vi "PID_2021.vi"(4 "Reset":bool, 5 "Lower limit":dbl, 6 "dt (s)":dbl, 7 "Upper limit":dbl, 8 "Setpoint":dbl, 9 "Process Variable":dbl, 10 "PID gains":cluster{"Kp":dbl, "Ki":dbl, "Kd":dbl}) -> (2 "u(t)":dbl)   [LabVIEW 2019]
panel:
  out "Error":dbl
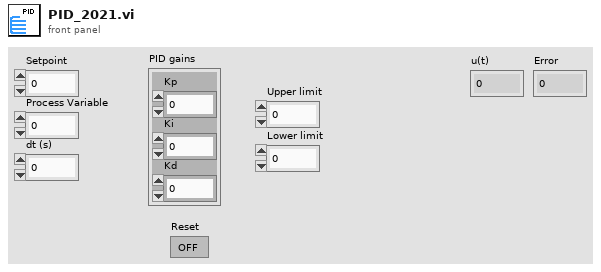
[diagram p1: front panel]
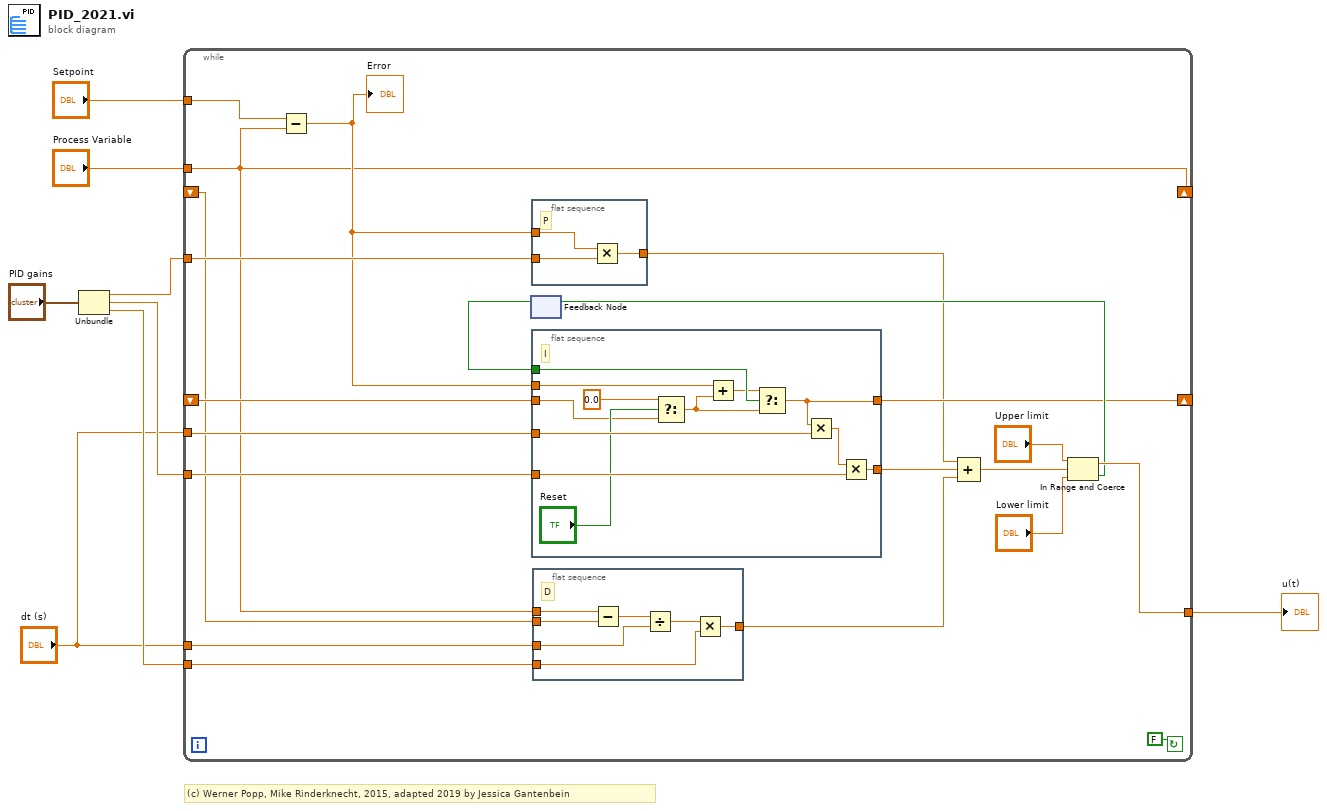
[diagram p0: block diagram]
diagram:
  # "(c) Werner Popp, Mike Rinderknecht, 2015, adapted 2019 by Jessica Gantenbein"
  n1 = Unbundle("PID gains") -> ("Kp"=w5:dbl, "Ki"=w4:dbl, "Kd"=w3:dbl)
  n2 = while {
    tunnel: "Setpoint" -> [w29]
    tunnel: "Process Variable" -> [w10]
    tunnel: w5 -> [w28]
    tunnel: w4 -> [w27]
    tunnel: w3 -> [w26]
    tunnel: "dt (s)" -> [w18]
    tunnel: "dt (s)" -> [w19]
    shift-right: [w14] -> _
    shift-left: _ -> [w13]
    tunnel: [w22] -> w1
    shift-right: [w10] -> _
    shift-left: _ -> [w9]
    stop <- FALSE continue-if-true
    n3 = Subtract(x=w29, y=w10) -> (x-y=w17:dbl)
    "Error" <- w17
    n4 = feedback #1() -> (w15:bool)  [unwired: 1 in]
    n5 = flat-sequence {
      tunnel: w17 -> [w51]
      tunnel: w28 -> [w50]
      tunnel: [w49] -> w12
      frame #0 {
        # "P"
        n6 = Multiply(x=w51, y=w50) -> (x*y=w49:dbl)
      }
    }
    n7 = flat-sequence {
      tunnel: w27 -> [w48]
      tunnel: [w47] -> w24
      tunnel: w19 -> [w45]
      tunnel: w17 -> [w38]
      tunnel: w15 -> [w44]
      tunnel: [w42] -> w14
      tunnel: w13 -> [w39]
      frame #0 {
        # "I"
        n8 = Select(t=0.0, s="Reset", f=w39) -> (s? t:f=w37:dbl)
        n9 = Add(x=w38, y=w37) -> (x+y=w43:dbl)
        n10 = Select(t=w43, s=w44, f=w37) -> (s? t:f=w42:dbl)
        n11 = Multiply(x=w42, y=w45) -> (x*y=w46:dbl)
        n12 = Multiply(x=w46, y=w48) -> (x*y=w47:dbl)
      }
    }
    n13 = flat-sequence {
      tunnel: w26 -> [w36]
      tunnel: [w35] -> w11
      tunnel: w18 -> [w34]
      tunnel: w10 -> [w33]
      tunnel: w9 -> [w30]
      frame #0 {
        # "D"
        n14 = Subtract(x=w33, y=w30) -> (x-y=w31:dbl)
        n15 = Divide(x=w31, y=w34) -> (x/y=w32:dbl)
        n16 = Multiply(x=w32, y=w36) -> (x*y=w35:dbl)
      }
    }
    n17 = Compound Arithmetic op=ADD(w12, w24, w11) -> (w23:dbl)
    n18 = In Range and Coerce(upper limit="Upper limit", x=w23, lower limit="Lower limit") -> (coerced(x)=w22:dbl, In Range?=w16:bool)
    n19 = feedback-in #1(w16) -> ()
  }
  "u(t)" <- w1
